vi "Vector2DArrayScale.vi"(9 "Scale":dbl, 11 "Vector Array":T1[](array[typedef])) -> (3 "Normalized Vector Array":T1[](array[typedef]))   [LabVIEW 2018]
uses:
  Vector2D.ctl
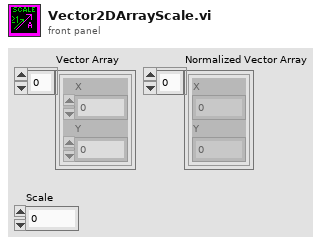
[diagram p1: front panel]
types:
  T1 = typedef "Vector2D.ctl" = cluster{"X":dbl, "Y":dbl}
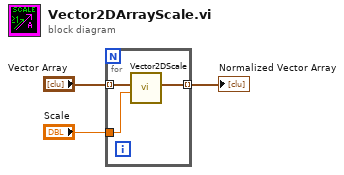
[diagram p0: block diagram]
diagram:
  n1 = for {
    tunnel: "Vector Array" -> [w6] mode=indexing
    tunnel: "Scale" -> [w5]
    tunnel: [w4] -> w1 mode=indexing
    n2 = call "Vector2DScale.vi"("Scale Factor"=w5, "Vector"=w6) -> ("Scaled Vector"=w4:T1)  [unwired: 9 in]
  }
  "Normalized Vector Array" <- w1
